vi "Gas_Setup.vi"() -> ()   [LabVIEW 2014]
uses:
  ADAM Controls/Ch_description_ADAM.ctl
  ADAM Controls/Module_type_ADAM.ctl
  ADAM Controls/Function_ADAM.ctl
  ADAM Controls/Channel_State.ctl
  ADAM Controls/Calib_type_ADAM.ctl
  ADAM Controls/Address.ctl
  ADAM Controls/Shut_Off_Valve.ctl
  ADAM Controls/Channel_names.ctl
  ADAM Controls/Update_scan_value.ctl
  Anemometry/Anemometry Sub Vis/Globals/Preference_global.vi
panel:
  out "Ch names":string[](array[string])
  in  "Select Plug Ins":bool
  in  "Source Info":string[][](table)
  in  "50 ml/min":T1
  in  "Carrier 1 Very Low":T1
  in  "Carrier 1 Hi-Tec Range":u16(ring) items=["Very Low", "Low", "High"]
  in  "Trace Hi-Tec Range":u16(ring) items=["5 ml/min", "50 ml/min", "300 ml/min"]
  in  "Carrier 1 High":T1
  in  "Carrier 1 Low":T1
  in  "300 ml/min":T1
  in  "5 ml/min":T1
  in  "Release Orientation":u16(ring) items=["Vertical", "Horizontal 0 Deg", "Downwards", "External System Tests", "Horizontal", "Edit Strings"]
  in  "Source Type":u16(ring) items=["11mm downward facing", "1mm Annulus above tank wall with Internal 2mm Annulus floating roof at 50mm.", "23mm IDD=8mm", "2mm Annulus around a quarter of inside of tank wall", "2mm Annulus around inside of tank wall", "4 point source ID=8.5mm located 90 deg apart on 8cm Diameter", "8mm Annulus around inside of tank wall", "B2 D=6.8mm", "B204 Height 244mm ID 5.5mm", "B230 Height 152.4mm ID 8.5mm", "B30 Area", "B311 ID=11mm", "B331 ID=5.4mm", "B38_8mm_ID_passive", "B38_OD=3.1mm_ID=2mm", "B548 OD=13.8mm ID=3.5mm", "D=12mm", "D=13.6mm", "D=16mm (ID=12 mm)", "D=18mm", "D=20mm", "D=22.5mm", "D=3.4mm", "D=5mm (ground release)", "D=6mm (ID=4.2 mm)", "D=7.1mm", "D=9mm", "D=9mm  20mm long passive", "Dext = 8.5 mm", "Exit Port of Solenoid Valve", "H=25:W=100mm", "H=50", "ID=15 mm 90 deg bend copper tube", "ID=5.1mm OD=5.8mm (Ground release)", "ID=5.1mm OD=5.8mm (roof release)", "ID=5mm OD=5.8mm", "ID=8.5mm OD=10mm", "ID=9.5mm OD=12.5mm", "Line Source 100mm  1.07m width", "Line Source 25mm  1.3m long  perp to flow", "Line Source 25x1300", "Line Source 50mm  1.07m Wide", "Line source parallel to flow", "None", "ROSE 9mm at last grid", "SAV ID=3.5mm", "Sample tubes in source", "Single 5mm Stack", "Single 7.9 mm stack", "THORP  ID=5.1mm", "Twin 5mm Stacks", "Twin Passive Stacks ID=8mm OD=8.7mm", "UKAEA ID=1.7mm", "W=50mm", "Edit Strings"]
  in  "Current Release Temp":dbl format="%.2f"
  in  "Release Temperature":u16(ring) items=["Enter Value", "EnFlo_Tunnel:Job:Name", "GMU:Source:Type", "GMU:Release:Orientation", "EnFlo_Tunnel:Obstacle/:Building", "EnFlo_Tunnel:Vorticity:Generators", "EnFlo_Tunnel:Roughness:Height", "EnFlo_Tunnel:Side Wall:Separation", "GMU:Trace:Gas", "GMU:Carrier 1:Gas", "GMU:Carrier 2:Gas", "GMU:Carrier 1:Hi-Tec Range", "GMU:Trace:Hi-Tec Range", "EnFlo_Tunnel:Obstacle:Orientation", "GMU:Source:Density Ratio", "GMU:Carrier 1:Dem Volt", "GMU:Carrier 2:Dem Volt", "GMU:Trace:Dem Volt", "GMU:Carrier 1:Meas Volt", "GMU:Carrier 2:Meas Volt", "GMU:Trace:Meas Volt", "GMU:Carrier 1:Meas Q", "GMU:Carrier 2:Meas Q", "GMU:Trace:Meas Q", "GMU:Carrier 1:Meas M_dot", "GMU:Carrier 2:Meas M_dot", "GMU:Trace:Meas M_dot", "GMU:Remaining:Nitrogen", "GMU:Remaining:Helium", "GMU:Remaining:CO2", "GMU:Remaining:Krypton", "GMU:Remaining:Ethane", "GMU:Remaining:Propane", "GMU:Calibration:Gas 1", "GMU:Calibration:Gas 2", "GMU:Signal FID:Calib Gas", "GMU:Source:Dem Q", "GMU:Source:Meas Q", "GMU:Source:Meas M_dot", "GMU:Source:Meas Density", "GMU:Source:Meas Den Ratio", "GMU:Source:Dem Strength", "GMU:Source:Meas Strength", "GMU:Source:Est Time", "GMU:Detector:Meas Current", "GMU:Detector:Strength", "Froude:NPL:Atmos_Press", "EnFlo Lab:Hygrometry:Rel Humidity", "EnFlo Lab:Hygrometry:Dew Point temp", "EnFlo Lab:Hygrometry:Air Temp", "GMU:Test:Ethane trip", "EnFlo_Tunnel:Safety:GMU_Watchdog", "EnFlo_Tunnel:Speed:Dem Velocity", "EnFlo_Tunnel:Speed:Calib Tweak", "EnFlo_Tunnel:Speed:Dem Current", "EnFlo_Tunnel:Usonic Fixed:Velocity", "EnFlo_Tunnel:Usonic Fixed:Direction", "EnFlo_Tunnel:Prop Y+ve:Velocity", "EnFlo_Tunnel:Prop Y-ve:Velocity", "EnFlo_Tunnel:Shaft:rpm", "EnFlo_Tunnel:Reference:Velocity", "EnFlo_Tunnel:Hydrosonic:Integral", "EnFlo_Tunnel:Days Run at:2.5m/s", "Hydrosonic:Transducer:Setting", "EnFlo_Tunnel:Trav Origin:X Offset", "EnFlo_Tunnel:Trav Pos:X", "EnFlo_Tunnel:Trav Pos:Y", "EnFlo_Tunnel:Trav Pos:Z", "EnFlo Lab:labstrat1:Z=4.5m", "EnFlo Lab:labstrat1:Z=3.5m", "EnFlo Lab:labstrat1:Z=2.5m", "EnFlo Lab:labstrat1:Z=1.5m", "EnFlo Lab:labstrat1:Z=0.5m", "EnFlo Lab:labstrat1:Delta T", "EnFlo Lab:Desired:Air Temp", "EnFlo Lab:Heat:Extraction", "EnFlo Lab:labstrat1:Av Temp", "University:Outside:Temp", "EnFlo_Tunnel:Inlet Heater:Temp 1", "EnFlo_Tunnel:Inlet Heater:Temp 2", "EnFlo_Tunnel:Inlet Heater:Temp 3", "EnFlo_Tunnel:Inlet Heater:Temp 4", "EnFlo_Tunnel:Inlet Heater:Temp 5", "EnFlo_Tunnel:Inlet Heater:Temp 6", "EnFlo_Tunnel:Inlet Heater:Temp 7", "EnFlo_Tunnel:Inlet Heater:Temp 8", "EnFlo_Tunnel:Inlet Heater:Temp 9", "EnFlo_Tunnel:Inlet Heater:Temp 10", "EnFlo_Tunnel:Inlet Heater:Temp 11", "EnFlo_Tunnel:Inlet Heater:Temp 12", "EnFlo_Tunnel:Inlet Heater:Temp 13", "EnFlo_Tunnel:Inlet Heater:Temp 14", "EnFlo_Tunnel:Inlet Heater:Temp 15", "EnFlo_Tunnel:Inlet Heater:Av Temp", "EnFlo_Tunnel:Inlet Heater:Max Temp", "EnFlo_Tunnel:Heater:Enable", "EnFlo_Tunnel:floor near:1", "EnFlo_Tunnel:floor near:3", "EnFlo_Tunnel:floor near:5", "EnFlo_Tunnel:floor far:7", "EnFlo_Tunnel:floor near:7", "EnFlo_Tunnel:floor far:9", "EnFlo_Tunnel:floor near:10", "EnFlo_Tunnel:floor near:11", "EnFlo_Tunnel:floor far:11", "EnFlo_Tunnel:Exit Duct:Temp", "EnFlo_Tunnel:Parker X:Temp", "EnFlo_Tunnel:roof near:19", "EnFlo_Tunnel:roof far:19", "EnFlo_Tunnel:Fan Gearbox:Y+ Temp", "EnFlo_Tunnel:Fan Gearbox:Y- Temp", "B_Tunnel:Motor:Temp", "Uni:Chilled Water:Temp", "EnFlo_Tunnel:Chilled Water:Motor1 Temp", "EnFlo_Tunnel:Chilled Water:Motor2 Temp", "EnFlo_Tunnel:Chilled Water:Supply", "EnFlo_Tunnel:Chilled Water:Return", "EnFlo_Tunnel:Chilled Water:Dem Temp", "EnFlo_Tunnel:Chilled Water:Valve Dem Pos", "EnFlo_Tunnel:Chilled Water:Valve Dem Voltage", "A_Tunnel:Trav:1", "A_Tunnel:Speed:Dem Velocity", "A_Tunnel:Speed:Calib Tweak", "A_Tunnel:Speed:Dem Voltage", "A_Tunnel:Motor:Temp", "GMU:Source:Release Temp", "Complete:Scan:Period", "D_Tunnel:Motor:Temp", "Cluster Room:General:Temp", "Cluster Room:Temp:Warning", "D_Tunnel:Speed:Dem Velocity", "D_Tunnel:Speed:Calib Tweak", "D_Tunnel:Speed:Dem Voltage", "EnFlo Lab:Underfloor Tank:Temp", "Laser:Cooling water:Return Temp", "EnFlo_Tunnel:User:Name", "A_Tunnel:User:Name", "D_Tunnel:User:Name", "Paul_Hayden:User:Name", "Uni:Chilled Water:Temp Warning", "Frauke_Desktop:User:Name", "ADAM_Server:User:Name", "Calibration_Tunnel:User:Name", "EnFlo_Tunnel:Side near:10", "EnFlo_Tunnel:Side far:10", "EnFlo_Tunnel:Source_Pos:X", "EnFlo_Tunnel:Source_Pos:Y", "EnFlo_Tunnel:Source_Pos:Z", "EnFlo_Tunnel:Max_Surface:Temp", "EnFlo_Tunnel:Chiller_Pump:Enable", "A_Tunnel:Motor:Enable", "GMU:Source:Divertor Valve", "EnFlo_Tunnel:Tap_Water:Enable", "EnFlo_Tunnel:Cooling_Panel:Manifold_Temp", "EnFlo_Tunnel:Motor:Enable", "EnFlo_Tunnel:Lights:Enable", "EnFlo_Tunnel:FFID:Temp", "GMU:Gas:Enable", "GMU:Detector:Happy", "EnFlo_Tunnel:Gas Solenoid:Status", "EnFlo_Tunnel:Usonic Inlet Z=75:Velocity", "EnFlo_Tunnel:Usonic Inlet Z=75:Direction", "GMU:Source:Pressure", "EnFlo_Tunnel:Wind:Direction", "Status:of:PB_G4_2", "PB_G4_2:User:Name", "EnFlo Lab:Comp Air:Pressure", "EnFlo Lab:Leak_Detector:Happy", "Paul_Desk:User:Name", "EnFlo Lab:Comp Air:Warning", "EnFlo_Tunnel:Turbine_1:Dem_Volts", "Laser:Cooling_Pump:Enable", "LDA:System:Enable", "FFID:System:Enable", "EnFlo_Tunnel:Motor:Temp", "Laser:Cooling water:Temp Warning", "GMU:Trace:Open", "No Match::", "EnFlo_Tunnel:Chiller_Pump:Running", "EnFlo_Tunnel:Parker X:Warning Temp", "B_Tunnel:User:Name", "EnFlo_Tunnel:Heat_Ex_Water:Return Temp", "EnFlo_Tunnel:Exit Duct Top:Temp", "LDA:3 Phase:Power", "Hydrosonic:Seeder:Enable", "Sugar:Water:Temp", "Hydrosonic:Tank:Temp", "A_Tunnel:Turbine:Enable", "A_Tunnel:Turbine_1:Dem_Volts"]
  in  "Gas Remaining":string[][](table)
  in  "Calib 2":dbl format="%.2f"
  in  "Calib 1":dbl format="%.2f"
  in  "Carrier 2 Gas":u16(ring) items=["Air", "Nitrogen", "Helium", "CO2", "Krypton", "None"]
  in  "Trace Gas":u16(ring) items=["Propane", "Ethane"]
  in  "Carrier 1 Gas":u16(ring) items=["Air", "Nitrogen", "Helium", "CO2", "Krypton", "None"]
  out "Numerical Values":dbl[](array[numeric]) format="%.9f"
  out "Ch Description Array":T2[](array[typedef]) {"Duty" format="%.0b"; "D" format="%#_5g"; "C" format="%#_5g"; "B" format="%#_5g"; "A" format="%#_5g"}
  out "dup reference":refnum<vi>
  in  "stop":bool
  in  "OK":bool
  # "Calibration Gas (ppm)"
  # "300\nml/min"
  # "5\nml/min"
  # "50\nml/min"
  # "Low\nRange"
  # "Very\nLow\nRange"
  # "High\nRange"
  # "Dispersion Setup"
  # "To Source"
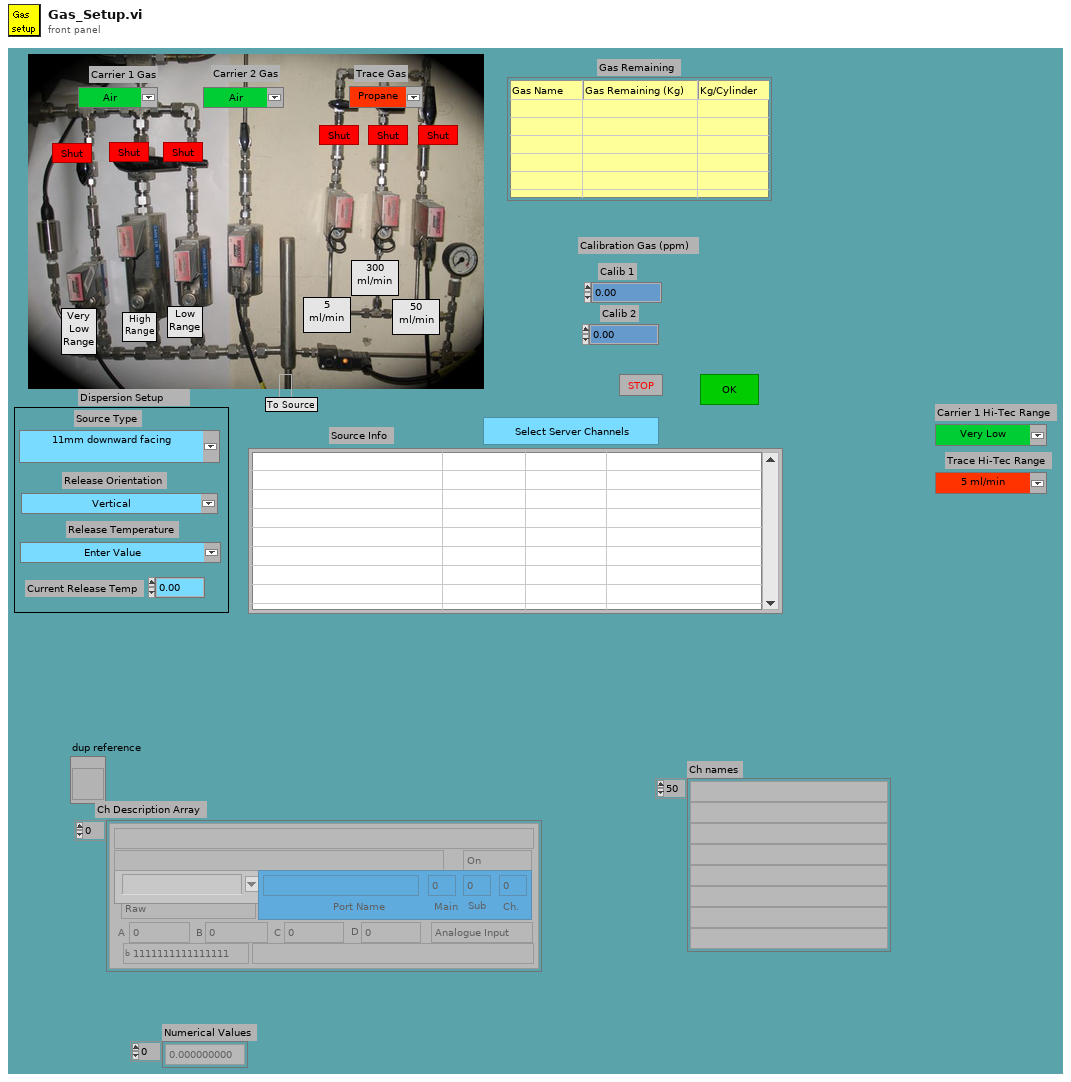
[diagram p1: front panel]
types:
  T1 = typedef "Shut_Off_Valve.ctl" = bool
  T2 = typedef "Ch_description_ADAM.ctl" = cluster{"Ch Name":string, "Type":T3, "Function":T4, "Ch State":T5, "Calibration type":T6, "A":dbl, "B":dbl, "C":dbl, "D":dbl, "Comments":string, "Address":T7, "String":string, "Duty":u16}
  T3 = typedef "Module_type_ADAM.ctl" = string
  T4 = typedef "Function_ADAM.ctl" = enum16{"Analogue Input", "Digital Input", "Event counter", "Event rate", "Analogue Output", "Digital Output", "Relay Output"}
  T5 = typedef "Channel_State.ctl" = enum16{"On", "Off", "Always On", "Always Off"}
  T6 = typedef "Calib_type_ADAM.ctl" = enum16{"Raw", "Bx + A", "Cx^2 + Bx + A", "Dx^3 + Cx^2 + Bx + A", "In Band", "Hi-Tec Q", "Hi-Tec M_dot", "Text"}
  T7 = typedef "Address.ctl" = cluster{"Main":i32, "Ch.":i32, "Sub":i32, "Port Name":string}
  T8 = typedef "Channel_names.ctl" = enum16{"Active Only", "Active + Off", "All Channels"}
  T9 = typedef "Update_scan_value.ctl" = cluster{"Channel Name":string, "New Value":dbl}
  T10 = enum16{"Zero or one", "One", "Zero or more", "One or more"}
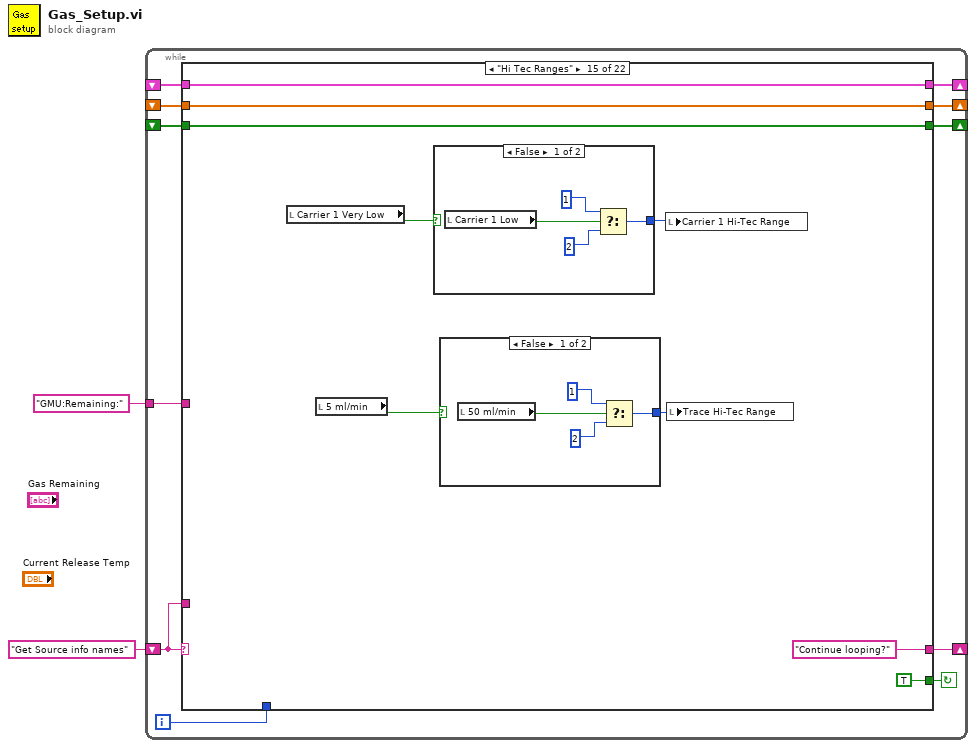
[diagram p0: block diagram]
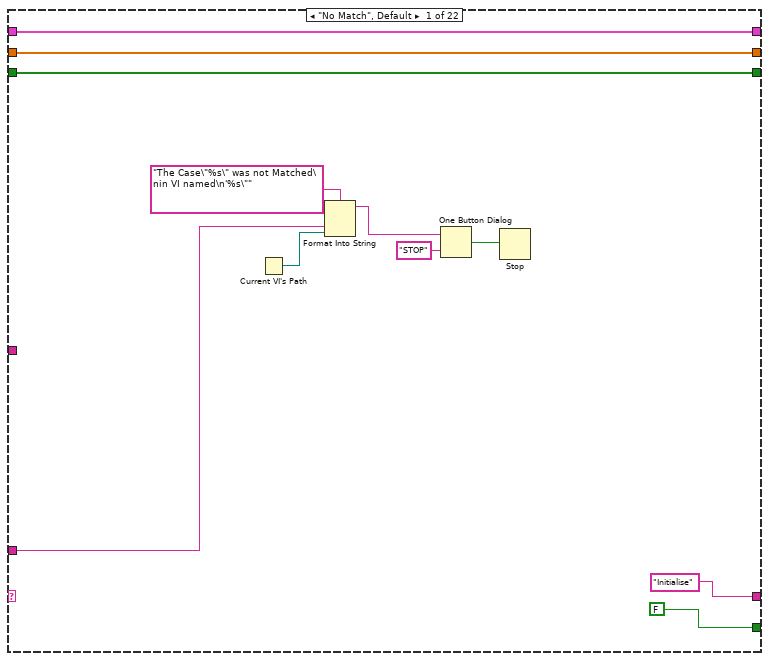
[diagram p2: hidden frame]
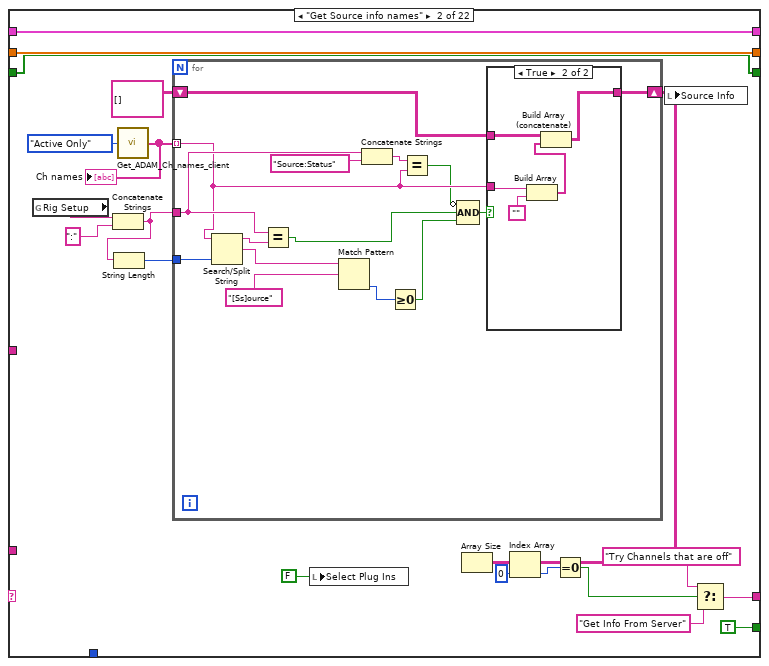
[diagram p3: hidden frame]
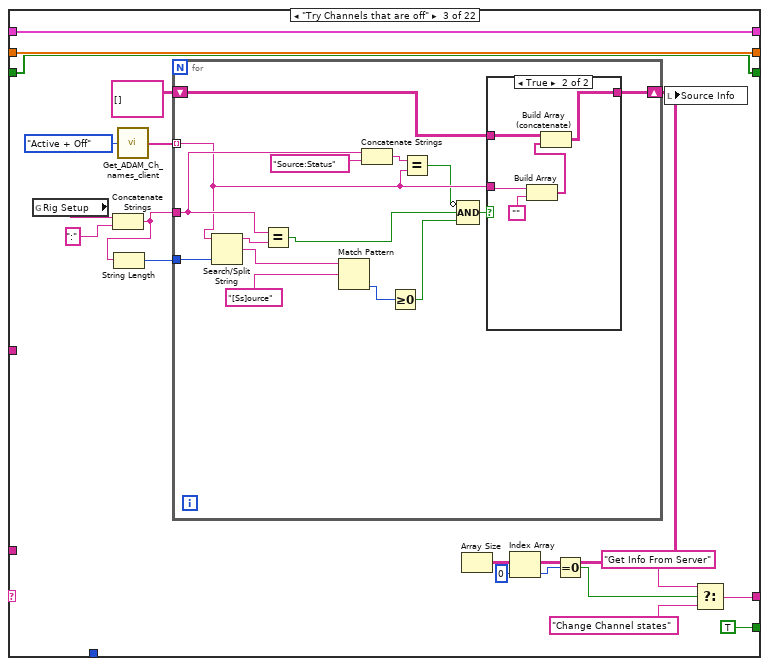
[diagram p5: hidden frame]
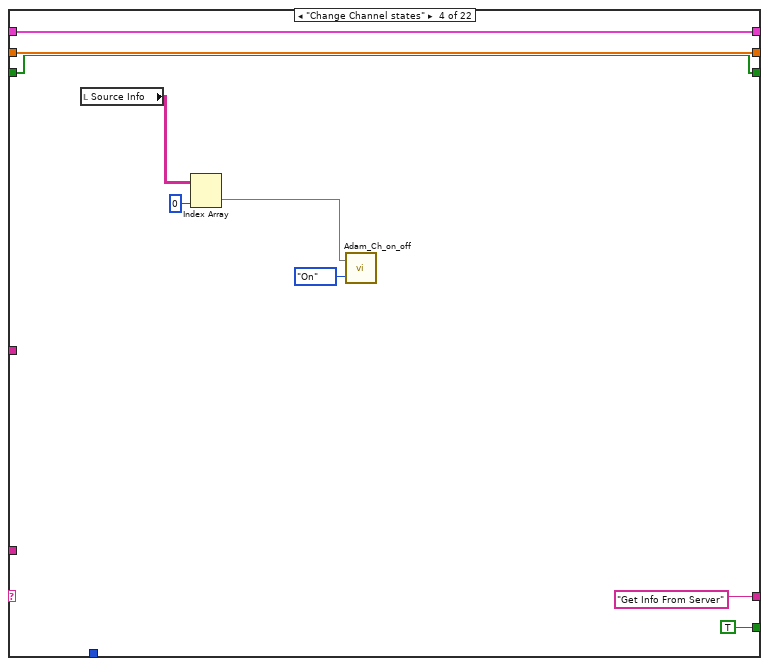
[diagram p7: hidden frame]
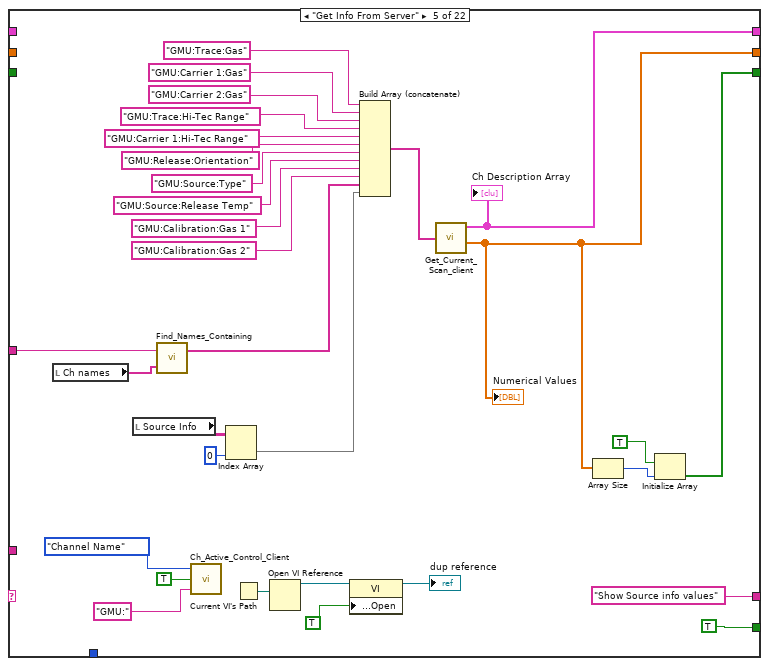
[diagram p8: hidden frame]
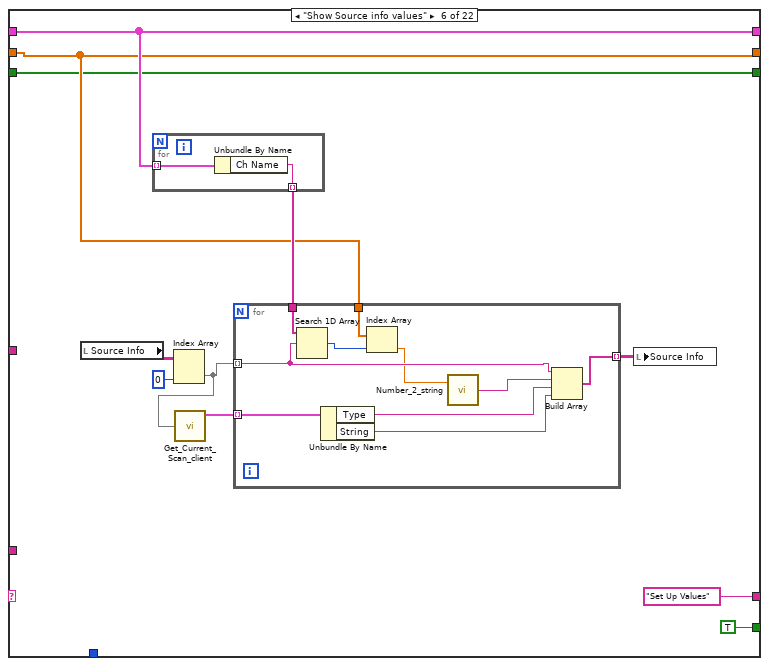
[diagram p9: hidden frame]
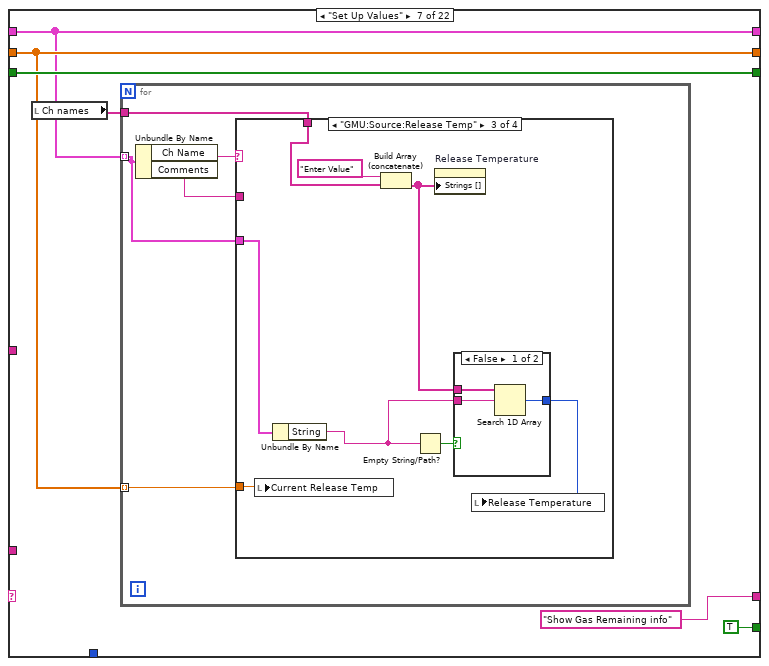
[diagram p10: hidden frame]
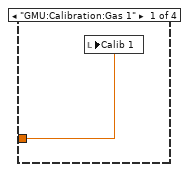
[diagram p11: hidden frame]
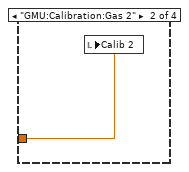
[diagram p12: hidden frame]
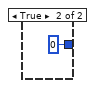
[diagram p13: hidden frame]
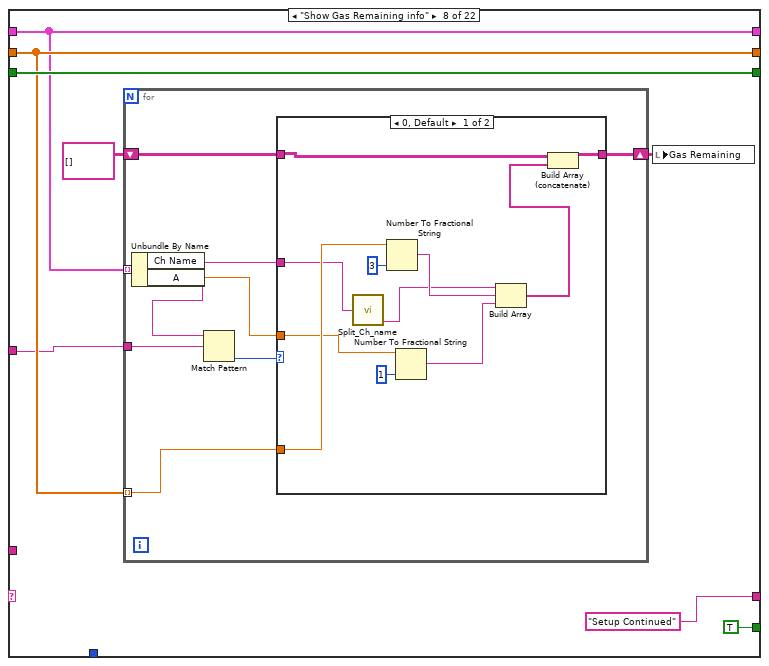
[diagram p15: hidden frame]
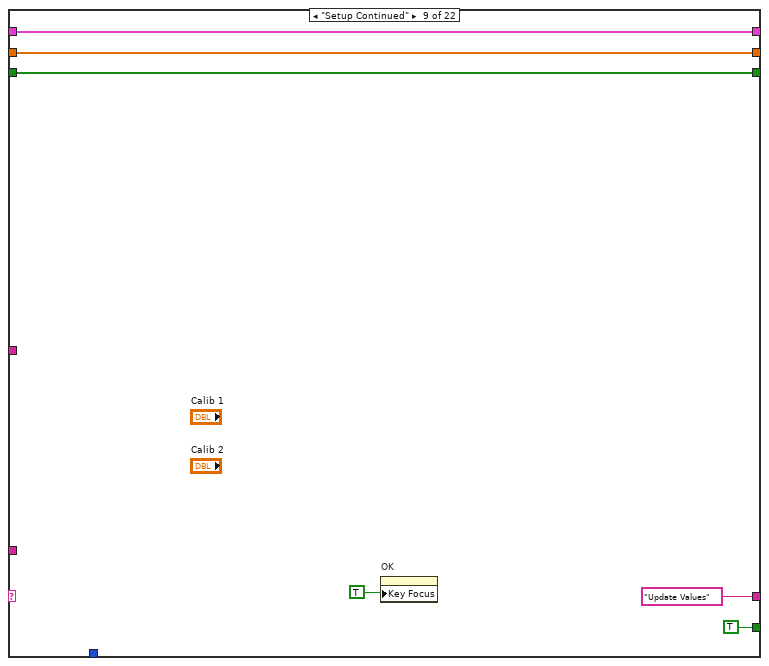
[diagram p17: hidden frame]
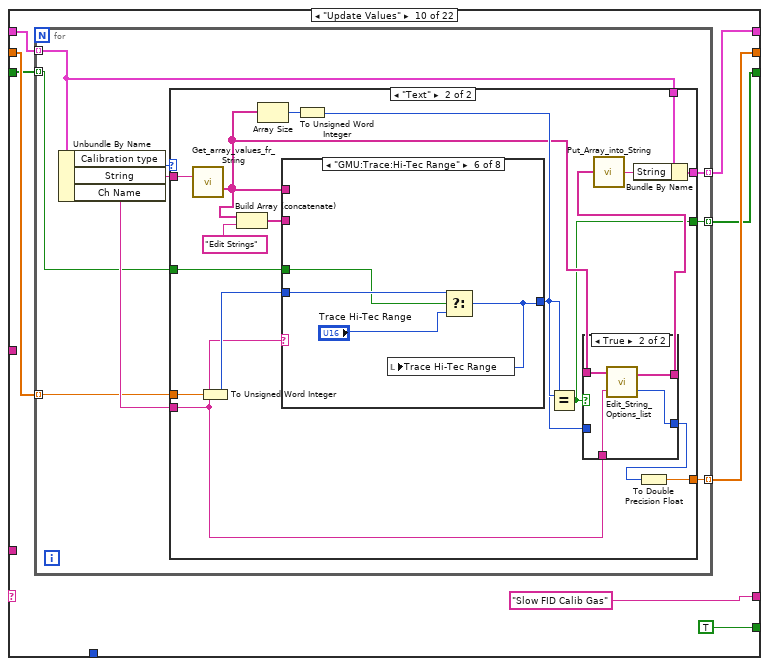
[diagram p18: hidden frame]
diagram:
  n1 = while {
    shift-left: _ -> [w5]
    shift-right: [w6] -> _
    shift-left: _ -> [w7]
    shift-right: [w9] -> _
    shift-left: _ -> [w8]
    shift-right: [w10] -> _
    shift-left: "Get Source info names" ("t") -> [w11]
    shift-right: [w12] -> _
    tunnel: "GMU:Remaining:" -> [w3]
    i -> [w4]
    stop <- w13 continue-if-true
    n2 = case shown="\"Hi Tec Ranges\"" w11 {
      tunnel: [FALSE TRUE ("T button?") TRUE ("T button?") TRUE ("T button?") TRUE TRUE ("T button?") TRUE ("T button?") TRUE ("T button?") TRUE ("T button?") TRUE ("T button?") TRUE ("T button?") TRUE ("T button?") TRUE ("T button?") TRUE ("T button?") TRUE ("T button?") TRUE ("T button?") TRUE ("T button?") TRUE ("T button?") TRUE ("T button?") TRUE ("T button?") TRUE ("T button?") FALSE ("T button?")] -> w13
      tunnel: ["Initialise" w26 w68 "Get Info From Server" "Show Source info values" "Set Up Values" "Show Gas Remaining info" "Setup Continued" "Update Values" "Slow FID Calib Gas" w311 "Update Release Temperature" "Sort out Valve Logic" "Hi Tec Ranges" "Continue looping?" w449 "Insert Gas Remaining Info" "Insert Source info values" "Update Server" w545 "Get Source info names" ("t") "End"] -> w12
      tunnel: w11 -> [w19 _ _ _ _ _ _ _ _ _ _ _ _ _ _ _ _ _ _ _ _ _]
      tunnel: [w16 w40 w80 w114 w138 w155 w170 w197 w227 w233 w315 w328 w358 w375 w433 w455 w457 w494 w526 w554 w610 w661] -> w10
      tunnel: [w15 w39 w79 w113 w125 w154 w171 w198 w226 w231 w314 w327 w357 w374 w432 w454 w460 w500 w528 w553 w609 w660] -> w9
      tunnel: w8 -> [w16 w40 w80 w114 _ w155 w170 w197 w227 w234 w315 w328 w358 w375 w433 w455 w458 w494 w526 w554 w610 w661]
      tunnel: w7 -> [w15 w39 w79 w113 _ w154 w171 w198 w226 w232 w314 w327 w357 w374 w432 w454 w459 w499 w529 w553 w609 w660]
      tunnel: [w14 w38 w78 w112 w124 w153 w173 w200 w224 w228 w309 w325 w355 w372 w430 w448 w462 w502 w525 w552 w608 w653] -> w6
      tunnel: w5 -> [w14 w38 w78 w112 _ w153 w173 w200 w224 w229 w309 w325 w355 w372 w430 w448 w462 w502 w525 w552 w608 w653]
      tunnel: w4 -> [_ _ _ _ _ _ _ _ _ _ w308 _ _ _ _ _ _ _ _ _ _ _]
      tunnel: w3 -> [_ _ _ _ w122 _ _ w196 _ _ _ _ _ _ _ _ _ w493 _ _ _ _]
      frame "No Match", Default {
        n3 = Current VI's Path() -> (path=w18:path)
        n4 = Format Into String(format string="The Case\"%s\" was not Matched\nin VI named\n'%s\"" ("Format String"), w19, w18) -> (resulting string=w22:string)  [unwired: 2 in, 1 out]
        n5 = One Button Dialog(message=w22, button name ("OK")="STOP") -> (true=w20:bool)
        n6 = Stop(stop? (T)=w20) -> ()
      }
      frame "Get Source info names" {
        n7 = global read "Preference_global.vi" "Rig Setup"() -> (w44:string)
        n8 = Concatenate Strings(w44, ":" ("string")) -> (w41:string)
        n9 = String Length(string=w41) -> (length=w42:i32)
        n10 = call "Get_ADAM_Ch_names_client.vi"("Channel names set"=Channel_names."Active Only") -> ("Ch names"=w35:string[])
        "Ch names" <- w35
        n11 = for {
          tunnel: w42 -> [w59]
          tunnel: w35 -> [w49] mode=indexing
          tunnel: w41 -> [w51]
          shift-right: [w53] -> w33
          shift-left: string[][] [] -> [w54]
          n12 = Search/Split String(string=w49, offset (0)=w59) -> (substring before match=w58:string, match + rest of string=w57:string)  [unwired: 2 out]
          n13 = Equal?(x=w51, y=w58) -> (x = y?=w47:bool)
          n14 = Match Pattern(string=w57, regular expression="[Ss]ource") -> (offset past match=w55:i32)  [unwired: 4 out]
          n15 = Concatenate Strings(w51, "Source:Status") -> (w50:string)
          n16 = Greater Or Equal To 0?(x=w55) -> (x >= 0?=w48:bool)
          n17 = Equal?(x=w50, y=w49) -> (x = y?=w46:bool)
          n18 = Compound Arithmetic op=AND(invert w46, w47, w48) -> (w45:bool)
          n19 = case shown="True" w45 {
            tunnel: w54 -> [w60 w65]
            tunnel: w49 -> [_ w63]
            tunnel: [w60 w64] -> w53
            frame False {
            }
            frame True {
              n20 = Build Array(w63, "") -> (w61:string[])
              n21 = Build Array (concatenate)(w65, w61) -> (w64:string[][])
            }
          }
        }
        n22 = local write "Select Plug Ins"(FALSE ("Select Plug Ins")) -> ()
        n23 = Array Size(array=w33) -> (size(s)=w32:i32[])
        n24 = Index Array(array=w32, index=0) -> (element=w30:i32)
        n25 = Equal To 0?(x=w30) -> (x = 0?=w28:bool)
        n26 = local write "Source Info"(w33) -> ()
        n27 = Select(t="Try Channels that are off", s=w28, f="Get Info From Server") -> (s? t:f=w26:string)
      }
      frame "Try Channels that are off" {
        n28 = global read "Preference_global.vi" "Rig Setup"() -> (w84:string)
        n29 = Concatenate Strings(w84, ":" ("string")) -> (w81:string)
        n30 = String Length(string=w81) -> (length=w82:i32)
        n31 = call "Get_ADAM_Ch_names_client.vi"("Channel names set"=Channel_names."Active + Off") -> ("Ch names"=w75:string[])
        n32 = for {
          tunnel: w82 -> [w99]
          tunnel: w75 -> [w89] mode=indexing
          tunnel: w81 -> [w91]
          shift-right: [w93] -> w74
          shift-left: string[][] [] -> [w94]
          n33 = Search/Split String(string=w89, offset (0)=w99) -> (substring before match=w98:string, match + rest of string=w97:string)  [unwired: 2 out]
          n34 = Equal?(x=w91, y=w98) -> (x = y?=w87:bool)
          n35 = Match Pattern(string=w97, regular expression="[Ss]ource") -> (offset past match=w95:i32)  [unwired: 4 out]
          n36 = Concatenate Strings(w91, "Source:Status") -> (w90:string)
          n37 = Greater Or Equal To 0?(x=w95) -> (x >= 0?=w88:bool)
          n38 = Equal?(x=w90, y=w89) -> (x = y?=w86:bool)
          n39 = Compound Arithmetic op=AND(invert w86, w87, w88) -> (w85:bool)
          n40 = case shown="True" w85 {
            tunnel: w94 -> [w100 w105]
            tunnel: w89 -> [_ w103]
            tunnel: [w100 w104] -> w93
            frame False {
            }
            frame True {
              n41 = Build Array(w103, "") -> (w101:string[])
              n42 = Build Array (concatenate)(w105, w101) -> (w104:string[][])
            }
          }
        }
        n43 = Array Size(array=w74) -> (size(s)=w73:i32[])
        n44 = Index Array(array=w73, index=0) -> (element=w71:i32)
        n45 = Equal To 0?(x=w71) -> (x = 0?=w69:bool)
        n46 = local write "Source Info"(w74) -> ()
        n47 = Select(t="Get Info From Server", s=w69, f="Change Channel states") -> (s? t:f=w68:string)
      }
      frame "Change Channel states" {
        n48 = local read "Source Info"() -> (w109:string[][])
        n49 = Index Array(array=w109, index (col)=0 ("disabled index (col)")) -> (element=w107:string[])  [unwired: 1 in]
        n50 = call "Adam_Ch_on_off.vi"("Ch State"=Channel_State."On", "ADAM Ch Names"=w107) -> ()  [unwired: 1 out]
      }
      frame "Get Info From Server" {
        n51 = local read "Ch names"() -> (w115:string[])
        n52 = local read "Source Info"() -> (w118:string[][])
        n53 = call "Find_Names_Containing.vi"("Ch names"=w115, "String to match"=w122) -> ("Matched Names"=w123:string[])  [unwired: 1 out]
        n54 = call "Ch_Active_Control_Client.vi"("Match"="GMU:", "Activate Channels?"=TRUE, "Control on"=enum16{"Channel Name", "Main Address"}."Channel Name") -> ()  [unwired: 2 out]
        n55 = Index Array(array=w118, index (col)=0 ("disabled index (col)")) -> (element=w116:string[])  [unwired: 1 in]
        n56 = Current VI's Path() -> (path=w140:path)
        n57 = Open VI Reference(vi path=w140) -> (vi reference=w141:refnum<vi>)  [unwired: 1 in, 5 out]
        n58 = property class="VI"(reference=w141, "Front Panel Window:Open"=TRUE) -> (reference out=→"dup reference":refnum<vi>)  [unwired: 1 in, 1 out]
        n59 = Build Array (concatenate)("GMU:Trace:Gas", "GMU:Carrier 1:Gas", "GMU:Carrier 2:Gas", "GMU:Trace:Hi-Tec Range", "GMU:Carrier 1:Hi-Tec Range", "GMU:Release:Orientation", "GMU:Source:Type", "GMU:Source:Release Temp", "GMU:Calibration:Gas 1", "GMU:Calibration:Gas 2", w123, w116) -> (w143:string[])
        n60 = call "Get_Current_Scan_client.vi"("ADAM Ch Names"=w143) -> ("Ch Description Array"=w138:T2[], "Numerical Values"=w125:dbl[])  [unwired: 2 out]
        "Ch Description Array" <- w138
        "Numerical Values" <- w125
        n61 = Array Size(array=w125) -> (size(s)=w127:i32)
        n62 = Initialize Array(TRUE, w127) -> (w124:bool[])
      }
      frame "Show Source info values" {
        n63 = local read "Source Info"() -> (w149:string[][])
        n64 = for {
          tunnel: w155 -> [w168] mode=indexing
          tunnel: [w167] -> w156 mode=indexing
          n65 = Unbundle By Name(w168) -> ("Ch Name"=w167:string)
        }
        n66 = Index Array(array=w149, index (col)=0 ("disabled index (col)")) -> (element=w147:string[])  [unwired: 1 in]
        n67 = call "Get_Current_Scan_client.vi"("ADAM Ch Names"=w147) -> ("Ch Description Array"=w146:T2[])  [unwired: 1 in, 2 out]
        n68 = for {
          tunnel: w156 -> [w166]
          tunnel: w147 -> [w163] mode=indexing
          tunnel: w154 -> [w164]
          tunnel: [w160] -> w152 mode=indexing
          tunnel: w146 -> [w159] mode=indexing
          n69 = Search 1D Array(1D array=w166, element=w163) -> (index of element=w165:i32)  [unwired: 1 out]
          n70 = Unbundle By Name(w159) -> ("Type"=w158:T3, "String"=w157:string)
          n71 = Index Array(array=w164, index=w165) -> (element=w162:dbl)
          n72 = call "Number_2_string.vi"("number"=w162) -> ("String"=w161:string)  [unwired: 1 in]
          n73 = Build Array(w163, w161, w158, w157) -> (w160:T3[])
        }
        n74 = local write "Source Info"(w152) -> ()
      }
      frame "Set Up Values" {
        n75 = local read "Ch names"() -> (w169:string[])
        n76 = for {
          tunnel: w171 -> [w175] mode=indexing
          tunnel: w170 -> [w177] mode=indexing
          tunnel: w169 -> [w176]
          n77 = Unbundle By Name(w177) -> ("Ch Name"=w179:string, "Comments"=w178:string)
          n78 = case shown="\"GMU:Source:Release Temp\"" w179 {
            tunnel: w175 -> [w180 w181 w185 _]
            tunnel: w178 -> [_ _ _ _]
            tunnel: w177 -> [_ _ w189 _]
            tunnel: w176 -> [_ _ w183 _]
            frame "GMU:Calibration:Gas 1" {
              n79 = local write "Calib 1"(w180) -> ()
            }
            frame "GMU:Calibration:Gas 2" {
              n80 = local write "Calib 2"(w181) -> ()
            }
            frame "GMU:Source:Release Temp" {
              n81 = local write "Current Release Temp"(w185) -> ()
              n82 = Unbundle By Name(w189) -> ("String"=w187:string)
              n83 = Build Array (concatenate)("Enter Value", w183) -> (w182:string[])
              n84 = Empty String/Path?(string/path=w187) -> (empty?=w188:bool)
              n85 = property on="Release Temperature" class="Ring (strict)"("Strings []"=w182) -> ()  [unwired: 2 in, 2 out]
              n86 = case shown="False" w188 {
                tunnel: w182 -> [w192 _]
                tunnel: w187 -> [w191 _]
                tunnel: [w190 0 ("index of element")] -> w186
                frame False {
                  n87 = Search 1D Array(1D array=w192, element=w191) -> (index of element=w190:i32)  [unwired: 1 out]
                }
                frame True {
                }
              }
              n88 = local write "Release Temperature"(w186) -> ()
            }
            frame "No Match", Default {
            }
          }
        }
      }
      frame "Show Gas Remaining info" {
        n89 = for {
          tunnel: w198 -> [w204] mode=indexing
          tunnel: w197 -> [w209] mode=indexing
          tunnel: w196 -> [w208]
          shift-right: [w205] -> w194
          shift-left: string[][] [] -> [w206]
          n90 = Unbundle By Name(w209) -> ("Ch Name"=w202:string, "A"=w203:dbl)
          n91 = Match Pattern(string=w202, regular expression=w208) -> (offset past match=w207:i32)  [unwired: 4 out]
          n92 = case shown="0, Default" w207 {
            tunnel: w206 -> [w211 w221]
            tunnel: [w210 w221] -> w205
            tunnel: w204 -> [w215 _]
            tunnel: w203 -> [w214 _]
            tunnel: w202 -> [w213 _]
            frame 0, Default {
              n93 = call "Split_Ch_name.vi"("Ch name"=w213) -> ("Low level"=w217:string)  [unwired: 2 out]
              n94 = Number To Fractional String(number=w215, precision (6)=i16 3) -> (F-format string=w220:string)  [unwired: 2 out]
              n95 = Number To Fractional String(number=w214, precision (6)=i16 1) -> (F-format string=w218:string)  [unwired: 2 out]
              n96 = Build Array(w217, w220, w218) -> (w212:string[])
              n97 = Build Array (concatenate)(w211, w212) -> (w210:string[][])
            }
            frame -1 {
            }
          }
        }
        n98 = local write "Gas Remaining"(w194) -> ()
      }
      frame "Setup Continued" {
        n99 = property on="OK" class="Bool"("Key Focus"=TRUE ("Write Attribute")) -> ()  [unwired: 2 in, 2 out]
      }
      frame "Update Values" {
        n100 = for {
          tunnel: w234 -> [w241] mode=indexing
          tunnel: [w240] -> w233 mode=indexing
          tunnel: w232 -> [w239] mode=indexing
          tunnel: [w238] -> w231 mode=indexing
          tunnel: w229 -> [w237] mode=indexing
          tunnel: [w236] -> w228 mode=indexing
          n101 = Unbundle By Name(w241) -> ("Calibration type"=w244:T6, "String"=w243:string, "Ch Name"=w242:string)
          n102 = case shown="\"Text\"" w244 {
            tunnel: w243 -> [_ w265]
            tunnel: w242 -> [_ w255]
            tunnel: w241 -> [w247 w259]
            tunnel: [w247 w258] -> w240
            tunnel: w239 -> [w246 w257]
            tunnel: [w246 w256] -> w238
            tunnel: w237 -> [w245 w254]
            tunnel: [w245 w248] -> w236
            frame "Raw", Default {
            }
            frame "Text" {
              n103 = call "Get_array_values_fr_String.vi"("String Value"=w265) -> ("String array"=w252:string[])  [unwired: 1 out]
              n104 = To Unsigned Word Integer(number=w257) -> (unsigned 16bit integer=w263:u16)
              n105 = Build Array (concatenate)(w252, "Edit Strings") -> (w251:string[])
              n106 = Array Size(array=w252) -> (size(s)=w264:i32)
              n107 = case shown="\"GMU:Trace:Hi-Tec Range\"" w255 {
                tunnel: [w272 w276 w281 w286 w290 w294 w299 w304] -> w249
                tunnel: w252 -> [_ w274 w278 w284 _ _ _ _]
                tunnel: w263 -> [w272 w277 w282 w287 w291 w295 w300 w305]
                tunnel: w254 -> [_ w275 w280 w285 w289 w293 w298 w303]
                tunnel: w251 -> [_ _ _ _ _ _ w297 w302]
                frame "No match", Default {
                }
                frame "GMU:Trace:Gas" {
                  n108 = property on="Trace Gas" class="Ring (strict)"("Strings []"=w274) -> ()  [unwired: 2 in, 2 out]
                  n109 = Select(t=w277, s=w275, f="Trace Gas") -> (s? t:f=w276:u16)
                  n110 = local write "Trace Gas"(w276) -> ()
                }
                frame "GMU:Carrier 1:Gas" {
                  n111 = property on="Carrier 1 Gas" class="Ring (strict)"("Strings []"=w278) -> ()  [unwired: 2 in, 2 out]
                  n112 = Select(t=w282, s=w280, f="Carrier 1 Gas") -> (s? t:f=w281:u16)
                  n113 = local write "Carrier 1 Gas"(w281) -> ()
                }
                frame "GMU:Carrier 2:Gas" {
                  n114 = property on="Carrier 2 Gas" class="Ring (strict)"("Strings []"=w284) -> ()  [unwired: 2 in, 2 out]
                  n115 = Select(t=w287, s=w285, f="Carrier 2 Gas") -> (s? t:f=w286:u16)
                  n116 = local write "Carrier 2 Gas"(w286) -> ()
                }
                frame "GMU:Carrier 1:Hi-Tec Range" {
                  n117 = Select(t=w291, s=w289, f="Carrier 1 Hi-Tec Range") -> (s? t:f=w290:u16)
                  n118 = local write "Carrier 1 Hi-Tec Range"(w290) -> ()
                }
                frame "GMU:Trace:Hi-Tec Range" {
                  n119 = Select(t=w295, s=w293, f="Trace Hi-Tec Range") -> (s? t:f=w294:u16)
                  n120 = local write "Trace Hi-Tec Range"(w294) -> ()
                }
                frame "GMU:Source:Type" {
                  n121 = property on="Source Type" class="Ring (strict)"("Strings []"=w297) -> ()  [unwired: 2 in, 2 out]
                  n122 = Select(t=w300, s=w298, f="Source Type") -> (s? t:f=w299:u16)
                  n123 = local write "Source Type"(w299) -> ()
                }
                frame "GMU:Release:Orientation" {
                  n124 = property on="Release Orientation" class="Ring (strict)"("Strings []"=w302) -> ()  [unwired: 2 in, 2 out]
                  n125 = Select(t=w305, s=w303, f="Release Orientation") -> (s? t:f=w304:u16)
                  n126 = local write "Release Orientation"(w304) -> ()
                }
              }
              n127 = To Unsigned Word Integer(number=w264) -> (unsigned 16bit integer=w262:u16)
              n128 = Equal?(x=w262, y=w249) -> (x = y?=w248:bool)
              n129 = case shown="True" w248 {
                tunnel: w252 -> [w267 w271]
                tunnel: w255 -> [_ w270]
                tunnel: [w267 w269] -> w260
                tunnel: [w266 w268] -> w250
                tunnel: w249 -> [w266 _]
                frame False {
                }
                frame True {
                  n130 = call "Edit_String_Options_list.vi"("Channel Name"=w270, "String array"=w271) -> ("New Selection Index"=w268:i32, "String array Out"=w269:string[])
                }
              }
              n131 = call "Put_Array_into_String.vi"("String array"=w260) -> ("String Value"=w261:string)
              n132 = Bundle By Name(cluster=w259, "String"=w261) -> (w258:T2)
              n133 = To Double Precision Float(number=w250) -> (double precision float=w256:dbl)
            }
          }
        }
      }
      frame "Slow FID Calib Gas" {
        n134 = Less?(x=w308, y=10) -> (x < y?=w306:bool)
        n135 = Select(t="Initialise Hi tec selection", s=w306, f="Update Release Temperature") -> (s? t:f=w311:string)
      }
      frame "Initialise Hi tec selection" {
        n136 = local read "Carrier 1 Hi-Tec Range"() -> (w323:u16)
        n137 = local read "Trace Hi-Tec Range"() -> (w319:u16)
        n138 = case shown="2" w323 {
          tunnel: [FALSE FALSE TRUE] -> w322
          tunnel: [FALSE TRUE FALSE] -> w321
          tunnel: [TRUE FALSE FALSE] -> w320
          frame 0, Default {
          }
          frame 1 {
          }
          frame 2 {
          }
        }
        n139 = case shown="0, Default" w319 {
          tunnel: [TRUE FALSE FALSE] -> w318
          tunnel: [FALSE TRUE FALSE] -> w317
          tunnel: [FALSE FALSE TRUE] -> w316
          frame 0, Default {
          }
          frame 1 {
          }
          frame 2 {
          }
        }
        n140 = local write "Carrier 1 Very Low"(w320) -> ()
        n141 = local write "Carrier 1 High"(w322) -> ()
        n142 = local write "Carrier 1 Low"(w321) -> ()
        n143 = local write "300 ml/min"(w316) -> ()
        n144 = local write "5 ml/min"(w318) -> ()
        n145 = local write "50 ml/min"(w317) -> ()
      }
      frame "Update Release Temperature" {
        n146 = while {
          tunnel: [w361] -> w352
          shift-left: _ -> [w361]
          shift-right: [w362] -> w353
          stop <- FALSE continue-if-true
          n147 = Get Date/Time In Seconds() -> (seconds since 1Jan1904=w359:timestamp)
          n148 = To Double Precision Float(number=w359) -> (double precision float=w362:dbl)
        }
        n149 = local read "Ch names"() -> (w347:string[])
        n150 = Not Equal To 0?(x="Release Temperature") -> (x != 0?=w350:bool)
        n151 = Not Equal?(x=w352, y=w353) -> (x != y?=w351:bool)
        n152 = And(x=w350, y=w351) -> (x .and. y?=w349:bool)
        n153 = case shown="True" w349 {
          tunnel: w347 -> [_ w365]
          tunnel: "Release Temperature" -> [_ w364]
          frame False {
          }
          frame True {
            n154 = Decrement(x=w364) -> (x-1=w363:u16)
            n155 = Index Array(array=w365, index=w363) -> (element=w370:string)
            n156 = Build Array(w370) -> (w369:string[])
            n157 = call "Get_Current_Scan_client.vi"("ADAM Ch Names"=w369) -> ("Numerical Values"=w367:dbl[])  [unwired: 3 out]
            n158 = Index Array(array=w367, index=0) -> (element=w366:dbl)
            n159 = local write "Current Release Temp"(w366) -> ()
          }
        }
      }
      frame "Sort out Valve Logic" {
        n160 = while {
          shift-left: _ -> [w378]
          shift-right: [w377] -> _
          shift-left: _ -> [w379]
          shift-right: [w380] -> _
          shift-left: _ -> [w381]
          shift-right: [w384] -> _
          shift-left: _ -> [w382]
          shift-right: [w383] -> _
          shift-left: _ -> [w385]
          shift-right: [w387] -> _
          shift-left: _ -> [w386]
          shift-right: [w388] -> _
          stop <- FALSE continue-if-true
          n161 = stacked-sequence {
            tunnel: ["Carrier 1 High" _] -> w388
            tunnel: ["Carrier 1 Low" _] -> w387
            tunnel: w386 -> [w397 _]
            tunnel: w385 -> [w396 _]
            tunnel: [_ "300 ml/min"] -> w384
            tunnel: [_ "5 ml/min"] -> w383
            tunnel: w382 -> [_ w411]
            tunnel: w381 -> [_ w410]
            tunnel: ["Carrier 1 Very Low" _] -> w380
            tunnel: w379 -> [w391 _]
            tunnel: w378 -> [_ w412]
            tunnel: [_ "50 ml/min"] -> w377
            frame #0 {
              n162 = Build Array("Carrier 1 Very Low", "Carrier 1 High", "Carrier 1 Low") -> (w395:T1[])
              n163 = Boolean To (0,1)(Boolean=w395) -> (0, 1=w394:i16[])
              n164 = Add Array Elements(numeric array=w394) -> (sum=w393:i16)
              n165 = case shown="2, Default" w393 {
                tunnel: w397 -> [_ _ w404]
                tunnel: w396 -> [_ _ w403]
                tunnel: "Carrier 1 Very Low" -> [_ _ w406]
                tunnel: w391 -> [_ _ w405]
                tunnel: "Carrier 1 Low" -> [_ _ w402]
                tunnel: "Carrier 1 High" -> [_ _ w401]
                frame 0 {
                }
                frame 1 {
                }
                frame 2, Default {
                  n166 = Exclusive Or(1:w405, 2:w406) -> (0:w400:T1)
                  n167 = Exclusive Or(1:w403, 2:w402) -> (0:w398:T1)
                  n168 = Exclusive Or(1:w404, 2:w401) -> (0:w399:T1)
                  n169 = local write "Carrier 1 Very Low"(w400) -> ()
                  n170 = local write "Carrier 1 High"(w399) -> ()
                  n171 = local write "Carrier 1 Low"(w398) -> ()
                }
              }
            }
            frame #1 {
              n172 = Build Array("50 ml/min", "5 ml/min", "300 ml/min") -> (w415:T1[])
              n173 = Boolean To (0,1)(Boolean=w415) -> (0, 1=w414:i16[])
              n174 = Add Array Elements(numeric array=w414) -> (sum=w413:i16)
              n175 = case shown="2, Default" w413 {
                tunnel: w411 -> [_ _ w422]
                tunnel: w410 -> [_ _ w421]
                tunnel: "50 ml/min" -> [_ _ w424]
                tunnel: w412 -> [_ _ w423]
                tunnel: "300 ml/min" -> [_ _ w420]
                tunnel: "5 ml/min" -> [_ _ w419]
                frame 0 {
                }
                frame 1 {
                }
                frame 2, Default {
                  n176 = Exclusive Or(1:w423, 2:w424) -> (0:w418:T1)
                  n177 = Exclusive Or(1:w421, 2:w420) -> (0:w416:T1)
                  n178 = Exclusive Or(1:w422, 2:w419) -> (0:w417:T1)
                  n179 = local write "300 ml/min"(w416) -> ()
                  n180 = local write "5 ml/min"(w417) -> ()
                  n181 = local write "50 ml/min"(w418) -> ()
                }
              }
            }
          }
        }
      }
      frame "Hi Tec Ranges" {
        n182 = local read "Carrier 1 Very Low"() -> (w426:T1)
        n183 = local read "5 ml/min"() -> (w427:T1)
        n184 = case shown="False" w426 {
          tunnel: [w436 u16 0 ("Carrier 1 Hi-Tec Range")] -> w425
          frame False {
            n185 = local read "Carrier 1 Low"() -> (w437:T1)
            n186 = Select(t=u16 1 ("Carrier 1 Hi-Tec Range"), s=w437, f=u16 2 ("Carrier 1 Hi-Tec Range")) -> (s? t:f=w436:u16)
          }
          frame True {
          }
        }
        n187 = case shown="False" w427 {
          tunnel: [w441 u16 0 ("Carrier 1 Hi-Tec Range")] -> w428
          frame False {
            n188 = local read "50 ml/min"() -> (w442:T1)
            n189 = Select(t=u16 1 ("Carrier 1 Hi-Tec Range"), s=w442, f=u16 2 ("Carrier 1 Hi-Tec Range")) -> (s? t:f=w441:u16)
          }
          frame True {
          }
        }
        n190 = local write "Carrier 1 Hi-Tec Range"(w425) -> ()
        n191 = local write "Trace Hi-Tec Range"(w428) -> ()
      }
      frame "Continue looping?" {
        n192 = local read "Select Plug Ins"() -> (w445:bool)
        n193 = Compound Arithmetic op=OR("stop", "OK", w445) -> (w444:bool)
        n194 = Current VI's Path() -> (path=w452:path)
        n195 = call "Close_Panel_and_Abort.vi"("Vi path"=w452, "stop"="stop") -> ()  [unwired: 1 out]
        n196 = Select(t="Insert Values", s=w444, f="Update Values") -> (s? t:f=w449:string)
      }
      frame "Insert Values" {
        n197 = local read "Ch names"() -> (w456:string[])
        n198 = for {
          tunnel: w458 -> [w466] mode=indexing
          tunnel: w459 -> [w468] mode=indexing
          tunnel: [w467] -> w460 mode=indexing
          tunnel: [w465] -> w457 mode=indexing
          tunnel: w456 -> [w464]
          n199 = Unbundle By Name(w466) -> ("Ch Name"=w469:string)
          n200 = case shown="\"GMU:Source:Release Temp\"" w469 {
            tunnel: w468 -> [_ _ _ w490]
            tunnel: [w470 w472 w474 w490] -> w467
            tunnel: w466 -> [w471 w473 w478 w489]
            tunnel: [w471 w473 w477 w489] -> w465
            tunnel: w464 -> [_ _ w476 _]
            frame "GMU:Calibration:Gas 1" {
              n201 = local read "Calib 1"() -> (w470:dbl)
            }
            frame "GMU:Calibration:Gas 2" {
              n202 = local read "Calib 2"() -> (w472:dbl)
            }
            frame "GMU:Source:Release Temp" {
              n203 = local read "Release Temperature"() -> (w475:u16)
              n204 = Equal To 0?(x=w475) -> (x = 0?=w481:bool)
              n205 = case shown="True" w481 {
                tunnel: w475 -> [w483 _]
                tunnel: w476 -> [w486 _]
                tunnel: [w485 ""] -> w479
                tunnel: [w484 w487] -> w480
                frame False {
                  w484 = T3 "Read Ch"  # Module Type
                  n206 = Decrement(x=w483) -> (x-1=w482:u16)
                  n207 = Index Array(array=w486, index=w482) -> (element=w485:string)
                }
                frame True {
                  w487 = T3 "Hold Value"  # Module Type
                }
              }
              n208 = local read "Current Release Temp"() -> (w474:dbl)
              n209 = Bundle By Name(cluster=w478, "String"=w479, "Type"=w480) -> (w477:T2)
            }
            frame "No Match", Default {
            }
          }
        }
      }
      frame "Insert Gas Remaining Info" {
        n210 = local read "Gas Remaining"() -> (w496:string[][])
        n211 = Index Array(array=w496, index (col)=0 ("disabled index (col)")) -> (element=w492:string[])  [unwired: 1 in]
        n212 = for {
          tunnel: w493 -> [w506]
          tunnel: w492 -> [w505] mode=indexing
          tunnel: [w504] -> w491 mode=indexing
          n213 = Concatenate Strings(w506, w505) -> (w504:string)
        }
        n214 = Index Array(array=w496, index (col)=1 ("disabled index (col)")) -> (element=w495:string[])  [unwired: 1 in]
        n215 = for {
          tunnel: w494 -> [w519] mode=indexing
          tunnel: w499 -> [w507] mode=indexing
          tunnel: [w515] -> w500 mode=indexing
          tunnel: w491 -> [w518]
          tunnel: w495 -> [w516]
          n216 = Unbundle By Name(w519) -> ("Ch Name"=w517:string)
          n217 = Search 1D Array(1D array=w518, element=w517) -> (index of element=w513:i32)  [unwired: 1 out]
          n218 = Number To Fractional String(number=w507, precision (6)=i16 3) -> (F-format string=w511:string)  [unwired: 2 out]
          n219 = Index Array(array=w516, index=w513) -> (element=w512:string)
          n220 = Greater Or Equal To 0?(x=w513) -> (x >= 0?=w510:bool)
          n221 = Not Equal?(x=w511, y=w512) -> (x != y?=w509:bool)
          n222 = And(x=w509, y=w510) -> (x .and. y?=w508:bool)
          n223 = case shown="False" w508 {
            tunnel: [w520 w522] -> w515
            tunnel: w512 -> [_ w521]
            tunnel: w507 -> [w520 _]
            frame False {
            }
            frame True {
              n224 = Fract/Exp String To Number(string=w521) -> (number=w522:dbl)  [unwired: 4 out]
            }
          }
        }
      }
      frame "Insert Source info values" {
        n225 = for {
          tunnel: w526 -> [w543] mode=indexing
          tunnel: [w542] -> w534 mode=indexing
          n226 = Unbundle By Name(w543) -> ("Ch Name"=w542:string)
        }
        n227 = Index Array(array="Source Info", index (col)=0 ("disabled index (col)")) -> (element=w530:string[])  [unwired: 1 in]
        n228 = Index Array(array="Source Info", index (col)=1 ("disabled index (col)")) -> (element=w527:string[])  [unwired: 1 in]
        n229 = for {
          tunnel: w534 -> [w541]
          tunnel: w530 -> [w540] mode=indexing
          shift-right: [w537] -> w528
          shift-left: w529 -> [w538]
          tunnel: w527 -> [w536] mode=indexing
          n230 = Fract/Exp String To Number(string=w536) -> (number=w535:dbl)  [unwired: 4 out]
          n231 = Search 1D Array(1D array=w541, element=w540) -> (index of element=w539:i32)  [unwired: 1 out]
          n232 = Replace Array Subset(array=w538, new element=w535, index=w539) -> (w537:dbl[])
        }
      }
      frame "Update Server" {
        w549 = T9 {"Channel Name"="", "New Value"=0.0} ("Update Scan Value Cluster")
        n233 = Index Array(array=w554, index=0 ("Index")) -> (element=w565:T2)
        n234 = local read "Ch Description Array"() -> (w551:T2[])
        n235 = local read "Numerical Values"() -> (w550:dbl[])
        n236 = Initialize Array(w565, 0 ("Dimension Size")) -> (w563:T2[])
        n237 = Initialize Array(w549, 0 ("Dimension Size")) -> (w558:T9[])
        n238 = for {
          shift-right: [w578] -> w560
          shift-left: w563 -> [w579]
          tunnel: w554 -> [w569] mode=indexing
          shift-right: [w577] -> w555
          shift-left: w558 -> [w576]
          tunnel: w553 -> [w571] mode=indexing
          tunnel: w551 -> [w570] mode=indexing
          tunnel: w550 -> [w574] mode=indexing
          tunnel: w549 -> [w572]
          n239 = Equal?(x=w569, y=w570) -> (x = y?=w575:bool)
          n240 = Equal?(x=w571, y=w574) -> (x = y?=w573:bool)
          n241 = case shown="False" w573 {
            tunnel: w576 -> [w586 w587]
            tunnel: [w585 w587] -> w577
            tunnel: w572 -> [w584 _]
            tunnel: w571 -> [w583 _]
            tunnel: w569 -> [w582 _]
            frame False {
              n242 = Unbundle By Name(w582) -> ("Ch Name"=w581:string)
              n243 = Bundle By Name(cluster=w584, "Channel Name"=w581, "New Value"=w583) -> (w580:T9)
              n244 = Build Array (concatenate)(w586, w580) -> (w585:T9[])
            }
            frame True {
            }
          }
          n245 = case shown="True" w575 {
            tunnel: w579 -> [w590 w591]
            tunnel: w569 -> [w589 _]
            tunnel: [w588 w591] -> w578
            frame False {
              n246 = Build Array (concatenate)(w590, w589) -> (w588:T2[])
            }
            frame True {
            }
          }
        }
        n247 = Array Size(array=w560) -> (size(s)=w562:i32)
        n248 = Array Size(array=w555) -> (size(s)=w556:i32)
        n249 = Greater Than 0?(x=w562) -> (x > 0?=w561:bool)
        n250 = Greater Than 0?(x=w556) -> (x > 0?=w557:bool)
        n251 = case shown="True" w561 {
          tunnel: w560 -> [_ w568]
          frame False {
          }
          frame True {
            n252 = call "Update_Ch_Discription_client.vi"("Channels to update In"=w568) -> ()  [unwired: 1 out]
          }
        }
        n253 = case shown="True" w557 {
          tunnel: w555 -> [_ w567]
          frame False {
          }
          frame True {
            n254 = call "Update_Current_Value_client.vi"("Update array in"=w567) -> ()  [unwired: 1 in]
          }
        }
        n255 = Select(t="Select Server Channels", s="Select Plug Ins", f="Close Panel") -> (s? t:f=w545:string)
      }
      frame "Select Server Channels" {
        w595 = string[] []
        w604 = T10."Zero or more"  # Selector mode
        n256 = local read "Source Info"() -> (w602:string[][])
        n257 = global read "Preference_global.vi" "Rig Setup"() -> (w615:string)
        n258 = Concatenate Strings(w615, ":" ("string")) -> (w612:string)
        n259 = String Length(string=w612) -> (length=w613:i32)
        n260 = call "Get_ADAM_Ch_names_client.vi"("Channel names set"=Channel_names."All Channels") -> ("Ch names"=w605:string[])
        n261 = Index Array(array=w602, index (col)=0) -> (element=w597:string[])  [unwired: 1 in]
        n262 = for {
          tunnel: w613 -> [w648]
          tunnel: w605 -> [w638] mode=indexing
          tunnel: w612 -> [w640]
          shift-right: [w642] -> w603
          shift-left: string[] [] -> [w643]
          n263 = Search/Split String(string=w638, offset (0)=w648) -> (substring before match=w647:string, match + rest of string=w646:string)  [unwired: 2 out]
          n264 = Equal?(x=w640, y=w647) -> (x = y?=w636:bool)
          n265 = Match Pattern(string=w646, regular expression="[Ss]ource") -> (offset past match=w644:i32)  [unwired: 4 out]
          n266 = Concatenate Strings(w640, "Source:Status") -> (w639:string)
          n267 = Greater Or Equal To 0?(x=w644) -> (x >= 0?=w637:bool)
          n268 = Equal?(x=w639, y=w638) -> (x = y?=w635:bool)
          n269 = Compound Arithmetic op=AND(invert w635, w636, w637) -> (w634:bool)
          n270 = case shown="True" w634 {
            tunnel: w643 -> [w649 w652]
            tunnel: w638 -> [_ w650]
            tunnel: [w649 w651] -> w642
            frame False {
            }
            frame True {
              n271 = Build Array (concatenate)(w652, w650) -> (w651:string[])
            }
          }
        }
        n272 = call "Select_Strings.vi"("Available Ch names"=w603, "Message"="Please select the appropriate source information channels", "Selector mode"=w604, "Desired Ch names (in)"=w597) -> ("Selected Channel Names"=w596:string[])  [unwired: 4 out]
        n273 = for {
          tunnel: w597 -> [w619] mode=indexing
          tunnel: w596 -> [w620]
          shift-right: [w616] -> w594
          shift-left: w595 -> [w617]
          n274 = Search 1D Array(1D array=w620, element=w619) -> (index of element=w618:i32)  [unwired: 1 out]
          n275 = case shown="-1" w618 {
            tunnel: w619 -> [_ w624]
            tunnel: w617 -> [w621 w623]
            tunnel: [w621 w622] -> w616
            frame 0, Default {
            }
            frame -1 {
              n276 = Build Array (concatenate)(w623, w624) -> (w622:string[])
            }
          }
        }
        n277 = call "Adam_Ch_on_off.vi"("Ch State"=Channel_State."Always Off", "ADAM Ch Names"=w594) -> ()  [unwired: 1 out]
        n278 = for {
          tunnel: w596 -> [w628] mode=indexing
          tunnel: w597 -> [w629]
          shift-right: [w625] -> w598
          shift-left: w595 -> [w626]
          n279 = Search 1D Array(1D array=w629, element=w628) -> (index of element=w627:i32)  [unwired: 1 out]
          n280 = case shown="-1" w627 {
            tunnel: w628 -> [_ w633]
            tunnel: w626 -> [w630 w632]
            tunnel: [w630 w631] -> w625
            frame 0, Default {
            }
            frame -1 {
              n281 = Build Array (concatenate)(w632, w633) -> (w631:string[])
            }
          }
        }
        n282 = call "Adam_Ch_on_off.vi"("Ch State"=Channel_State."On", "ADAM Ch Names"=w598) -> ()  [unwired: 1 out]
      }
      frame "Close Panel" {
        n283 = local read "dup reference"() -> (w654:refnum<vi>)
        n284 = property class="VI"(reference=w654, "Front Panel Window:Open"=FALSE) -> (reference out=w656:refnum<vi>, error out=w655:errorcluster)  [unwired: 1 in]
        n285 = Close Reference(reference=w656, error in (no error)=w655) -> ()  [unwired: 1 out]
      }
    }
  }
